vi "saveSensorsData.vi"(1 "SensorsData":T1(array[cluster]), 2 "file path (dialog if empty)":path) -> ()   [LabVIEW 2021]
uses:
  <vilib>/Utility/file.llb/Write Delimited Spreadsheet (string).vi
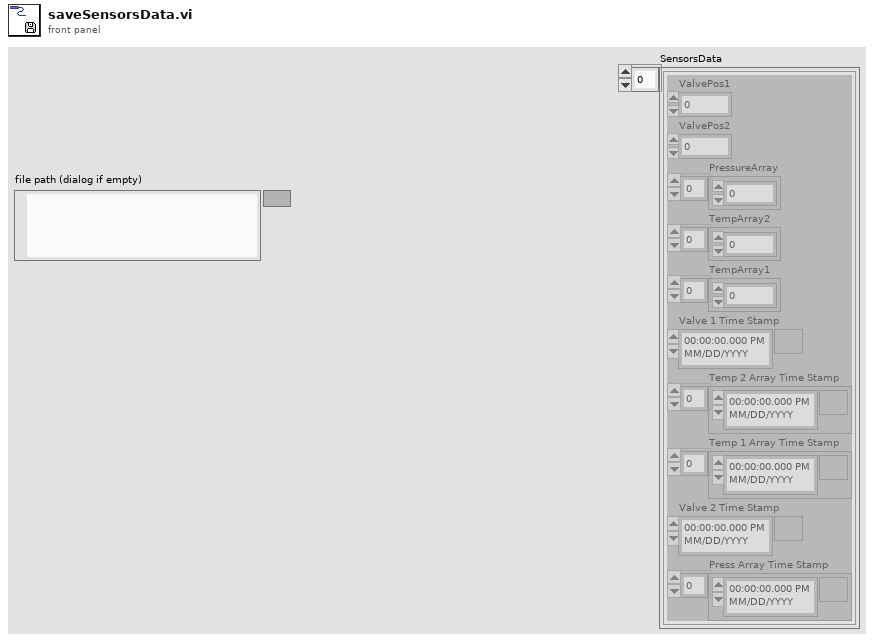
[diagram p1: front panel]
types:
  T1 = cluster{"ValvePos1":sgl, "ValvePos2":sgl, "PressureArray":sgl[], "TempArray2":sgl[], "TempArray1":sgl[], "Valve 1 Time Stamp":timestamp, "Temp 2 Array Time Stamp":timestamp[], "Temp 1 Array Time Stamp":timestamp[], "Valve 2 Time Stamp":timestamp, "Press Array Time Stamp":timestamp[]}[]
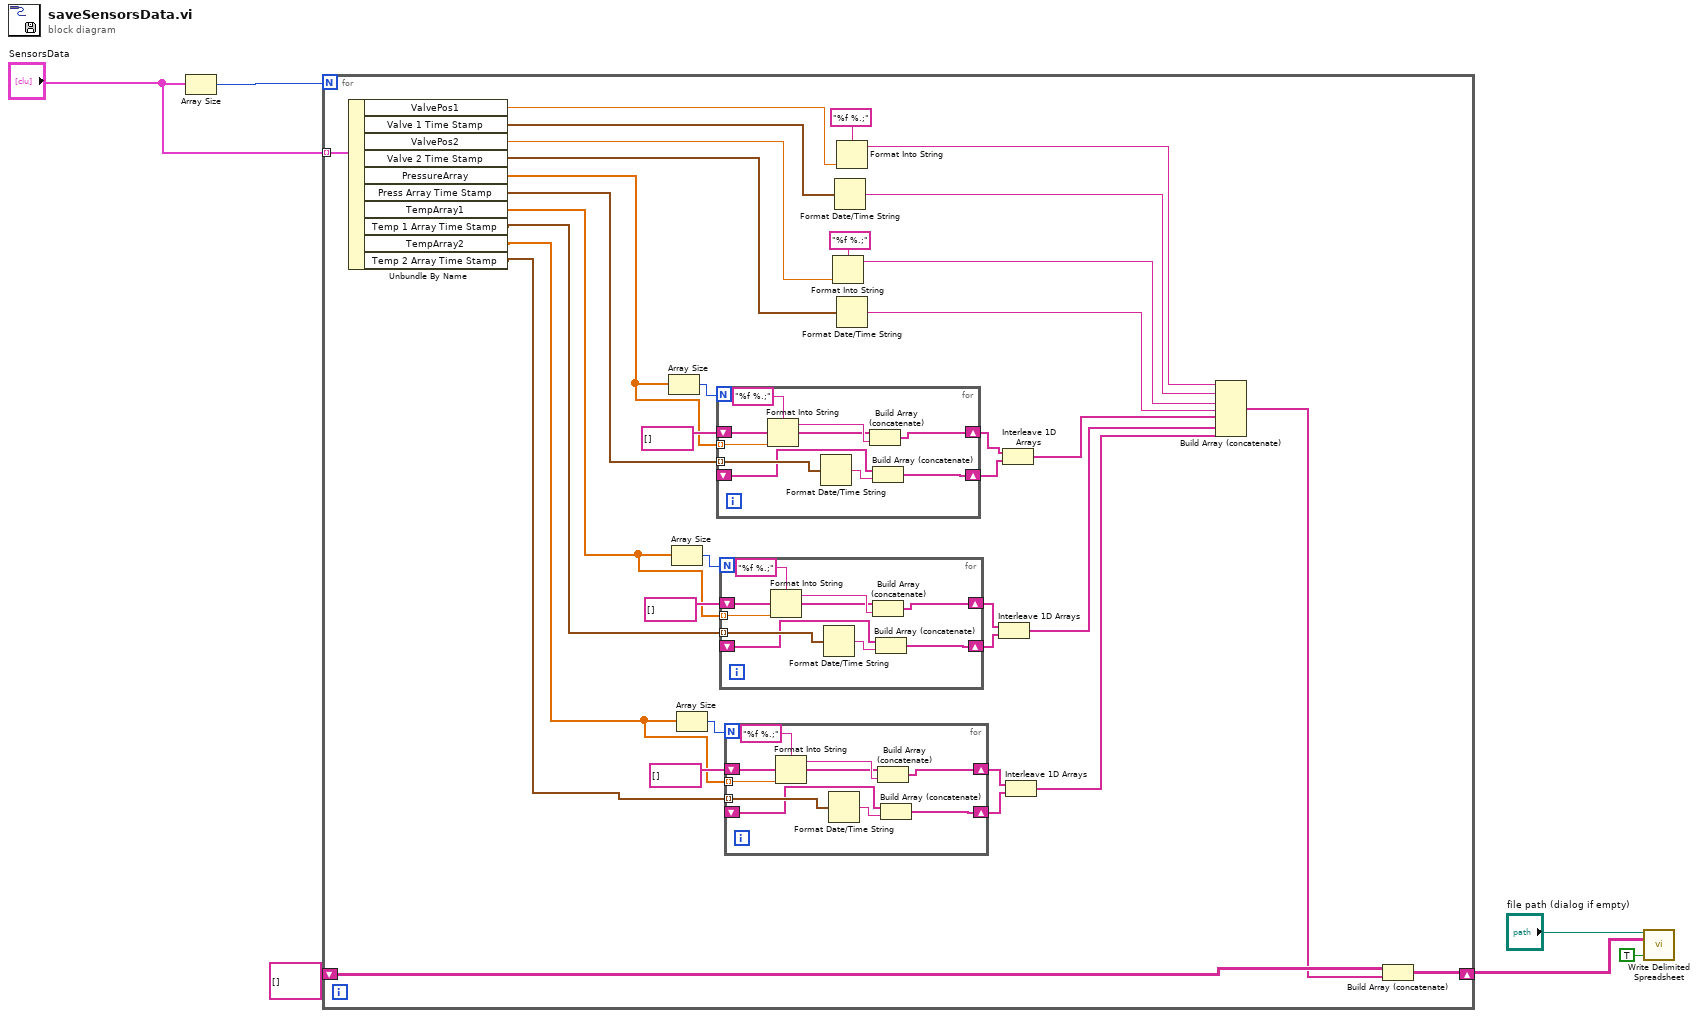
[diagram p0: block diagram]
diagram:
  n1 = Array Size(array="SensorsData") -> (size(s)=w6:i32)
  n2 = for {
    N: w6 -> [_]
    tunnel: "SensorsData" -> [w38] mode=indexing
    shift-right: [w16] -> w4
    shift-left: string[][] [] -> [w35]
    n3 = Unbundle By Name(w38) -> ("ValvePos1"=w37:sgl, "Valve 1 Time Stamp"=w34:timestamp, "ValvePos2"=w31:sgl, "Valve 2 Time Stamp"=w30:timestamp, "PressureArray"=w27:sgl[], "Press Array Time Stamp"=w26:timestamp[], "TempArray1"=w21:sgl[], "Temp 1 Array Time Stamp"=w20:timestamp[], "TempArray2"=w19:sgl[], "Temp 2 Array Time Stamp"=w18:timestamp[])
    n4 = Array Size(array=w27) -> (size(s)=w41:i32)
    n5 = Array Size(array=w21) -> (size(s)=w25:i32)
    n6 = Array Size(array=w19) -> (size(s)=w23:i32)
    n7 = for {
      N: w41 -> [_]
      shift-right: [w67] -> w15
      shift-left: string[] [] -> [w66]
      shift-right: [w61] -> w14
      shift-left: _ -> [w60]
      tunnel: w27 -> [w64] mode=indexing
      tunnel: w26 -> [w63] mode=indexing
      n8 = Format Into String(format string="%f %.;", w64) -> (resulting string=w68:string)  [unwired: 2 in, 1 out]
      n9 = Format Date/Time String(seconds (now)=w63) -> (date/time string=w62:string)  [unwired: 2 in]
      n10 = Build Array (concatenate)(w66, w68) -> (w67:string[])
      n11 = Build Array (concatenate)(w60, w62) -> (w61:string[])
    }
    n12 = for {
      N: w25 -> [_]
      shift-right: [w58] -> w13
      shift-left: string[] [] -> [w57]
      shift-right: [w52] -> w12
      shift-left: _ -> [w51]
      tunnel: w21 -> [w55] mode=indexing
      tunnel: w20 -> [w54] mode=indexing
      n13 = Format Into String(format string="%f %.;", w55) -> (resulting string=w59:string)  [unwired: 2 in, 1 out]
      n14 = Format Date/Time String(seconds (now)=w54) -> (date/time string=w53:string)  [unwired: 2 in]
      n15 = Build Array (concatenate)(w57, w59) -> (w58:string[])
      n16 = Build Array (concatenate)(w51, w53) -> (w52:string[])
    }
    n17 = for {
      N: w23 -> [_]
      shift-right: [w49] -> w11
      shift-left: string[] [] -> [w48]
      shift-right: [w43] -> w10
      shift-left: _ -> [w42]
      tunnel: w19 -> [w46] mode=indexing
      tunnel: w18 -> [w45] mode=indexing
      n18 = Format Into String(format string="%f %.;", w46) -> (resulting string=w50:string)  [unwired: 2 in, 1 out]
      n19 = Format Date/Time String(seconds (now)=w45) -> (date/time string=w44:string)  [unwired: 2 in]
      n20 = Build Array (concatenate)(w48, w50) -> (w49:string[])
      n21 = Build Array (concatenate)(w42, w44) -> (w43:string[])
    }
    n22 = Format Into String(format string="%f %.;", w31) -> (resulting string=w29:string)  [unwired: 2 in, 1 out]
    n23 = Format Date/Time String(seconds (now)=w34) -> (date/time string=w32:string)  [unwired: 2 in]
    n24 = Format Into String(format string="%f %.;", w37) -> (resulting string=w33:string)  [unwired: 2 in, 1 out]
    n25 = Format Date/Time String(seconds (now)=w30) -> (date/time string=w28:string)  [unwired: 2 in]
    n26 = Interleave 1D Arrays(w13, w12) -> (w8:string[])
    n27 = Interleave 1D Arrays(w15, w14) -> (w9:string[])
    n28 = Interleave 1D Arrays(w11, w10) -> (w7:string[])
    n29 = Build Array (concatenate)(w33, w32, w29, w28, w9, w8, w7) -> (w17:string[])
    n30 = Build Array (concatenate)(w35, w17) -> (w16:string[][])
  }
  n31 = call-poly <vilib>:"Write Delimited Spreadsheet.vi"("file path (dialog if empty)"="file path (dialog if empty)", "2D data"=w4, "append to file? (new file:F)"=TRUE) -> ()  [unwired: 11 in, 2 out]
